vi "AWGSwitchtoAFG.vi"(2 "error in (no error)":errorcluster, 3 "VISA resource name":refnum<visa-resource-name>) -> (0 "error out":errorcluster, 1 "VISA resource name out":refnum<visa-resource-name>)   [LabVIEW 2020, in "Active Technologies AWG3000.lvlib"]
uses:
  Active Technologies AWG3000.lvlib
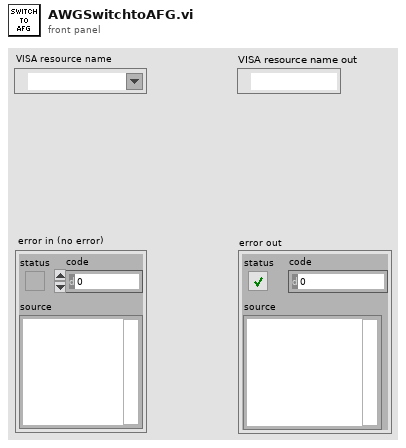
[diagram p1: front panel]
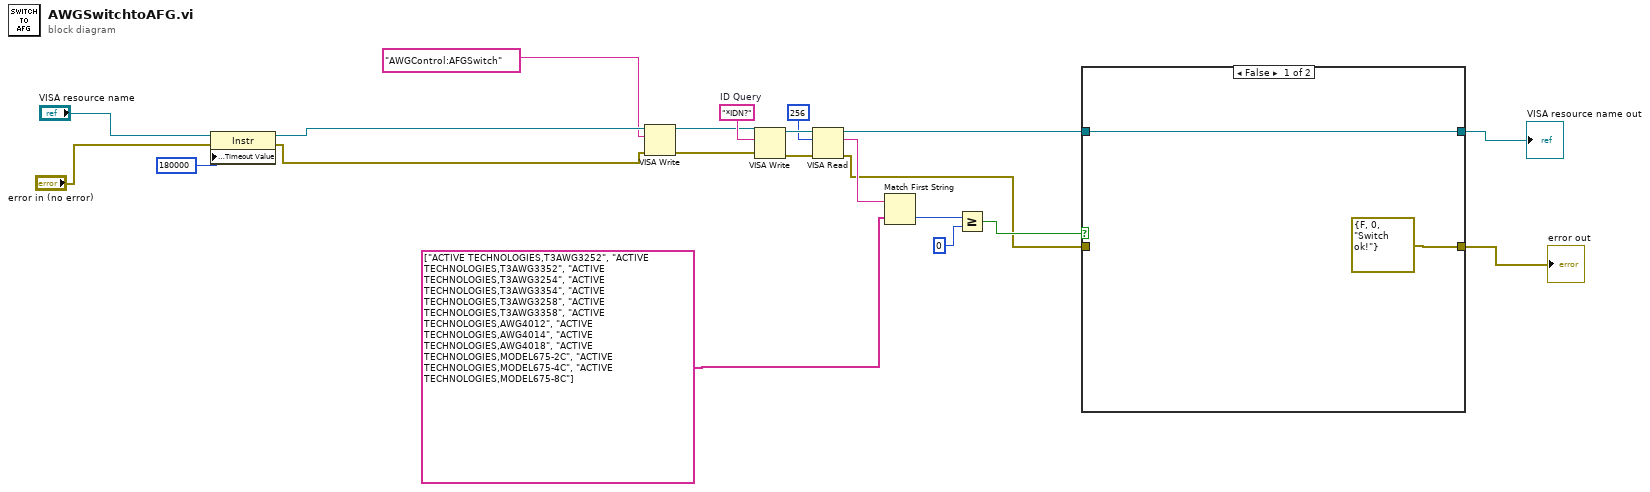
[diagram p0: block diagram]
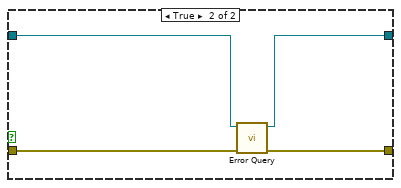
[diagram p2: hidden frame]
diagram:
  w14 = "*IDN?"  # ID Query
  n1 = property class="Instr"(reference="VISA resource name", error in="error in (no error)", "General Settings:Timeout Value"=u32 180000) -> (reference out=w18:refnum<visa-resource-name>, error out=w19:errorcluster)
  n2 = VISA Write(VISA resource name=w18, write buffer="AWGControl:AFGSwitch", error in (no error)=w19) -> (VISA resource name out=w4:refnum<visa-resource-name>, error out=w3:errorcluster)  [unwired: 1 out]
  n3 = VISA Write(VISA resource name=w4, write buffer=w14, error in (no error)=w3) -> (VISA resource name out=w17:refnum<visa-resource-name>, error out=w16:errorcluster)  [unwired: 1 out]
  n4 = VISA Read(VISA resource name=w17, byte count=u32 256, error in (no error)=w16) -> (VISA resource name out=w9:refnum<visa-resource-name>, read buffer=w13:string, error out=w8:errorcluster)  [unwired: 1 out]
  n5 = Match First String(2:string[] ["ACTIVE TECHNOLOGIES,T3AWG3252", "ACTIVE TECHNOLOGIES,T3AWG3352", "ACTIVE TECHNOLOGIES,T3AWG3254", "ACTIVE TECHNOLOGIES,T3AWG3354", "ACTIVE TECHNOLOGIES,T3AWG3258", "ACTIVE TECHNOLOGIES,T3AWG3358", "ACTIVE TECHNOLOGIES,AWG4012", "ACTIVE TECHNOLOGIES,AWG4014", "ACTIVE TECHNOLOGIES,AWG4018", "ACTIVE TECHNOLOGIES,MODEL675-2C", "ACTIVE TECHNOLOGIES,MODEL675-4C", "ACTIVE TECHNOLOGIES,MODEL675-8C"] ("reversed array"), 3:w13) -> (0:w12:i32)  [unwired: 1 out]
  n6 = Greater Or Equal?(x=w12, y=0) -> (x >= y?=w10:bool)
  n7 = case shown="False" w10 {
    tunnel: w9 -> [w23 w27]
    tunnel: w8 -> [_ w26]
    tunnel: [w23 w25] -> w7
    tunnel: [errorcluster {"status"=FALSE, "code"=0, "source"="Switch ok!"} ("error out") w24] -> w6
    frame False {
    }
    frame True {
      n8 = call "Error Query.vi"("error in (no error)"=w26, "VISA resource name"=w27) -> ("error out"=w24:errorcluster, "VISA resource name out"=w25:refnum<visa-resource-name>)  [unwired: 6 in, 2 out]
    }
  }
  "VISA resource name out" <- w7
  "error out" <- w6
